vi "SendCmdToSkywire.vi"(6 "wait for response (y)":bool=TRUE, 8 "error in (no error)":errorcluster, 9 "Cmd String":string="AT+CSQ", 10 "Cmd":T1=enum."Send cmd string", 11 "VISA resource name":refnum<visa-resource-name>="COM30") -> (0 "error out":errorcluster, 1 "Response numbers":dbl[](array[numeric])=[5.0, 3.0], 2 "Response string":string="AT+CSQ\r\r\n+CSQ: 5,3\r\n\r\nOK\r\n", 3 "VISA resource name 2":refnum<visa-resource-name>="COM30", 4 "Parsed string response":string, 5 "Parsed string responses":string[](array[string]), 7 "RSSI (dbm)":string="-103")   [LabVIEW 2013]
uses:
  Skywire cmds.ctl
  Test Globals/Global 1.vi
  Main Support/Global 2.vi
panel:
  out "Log resp":string
  out "Msecs to stopped":u32
  out "Msecs to first byte":u32
  out "Bytes at Port":u32=26
  out "timeout":bool
  out "return count":u32=7
  in  "CmdArray":string[](array[string])=["AT+CSQ", "AT+CGMR", "AT+CREG?", "AT+CGREG?", "AT#MEIDESN?", "AT+CGSN", "AT$GPSLOCK?", "In cmd string", "AT", "AT#SIMDET=1", "AT#HDRPS?", "AT+GMM", "AT+KSIMDET=1", "AT#CCID", "AT+CEREG?", "AT+CGMM", "AT+GSN", "AT#SIMDET?"]
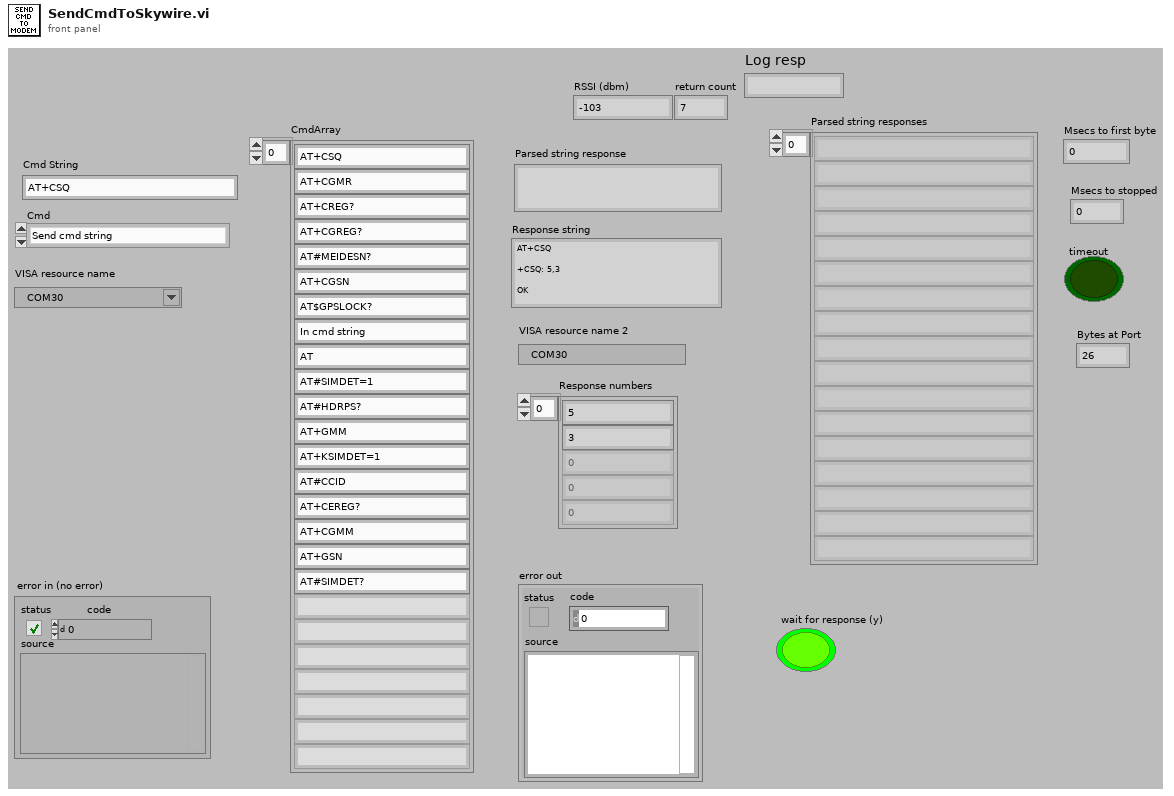
[diagram p1: front panel]
types:
  T1 = typedef "Skywire cmds.ctl" = enum16{"Get primary RSSI", "Get firmware version", "Check 2/3G network reception", "Check LTE network reception", "Get MEID for CDMA", "Get IMEI for 4G/LTE", "Get GPS Coordinates", "Send cmd string", "Check communications", "Enable sim detect", "Check diversity RSSI", "Get make model", "Sierra enable sim det", "get ccid sim id", "Get Gemalto Net Reg", "Get Gemalto model", "Get modem serial number", "Telit sim detect"}
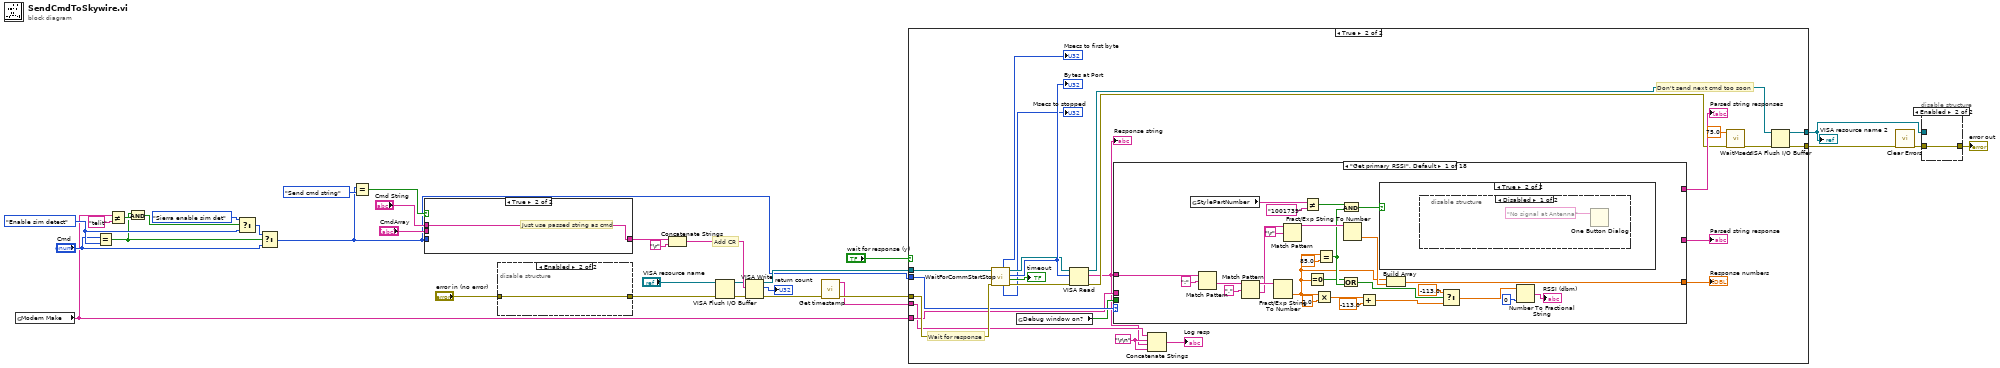
[diagram p0: block diagram]
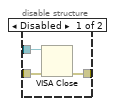
[diagram p2: hidden frame]
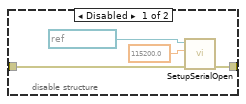
[diagram p3: hidden frame]
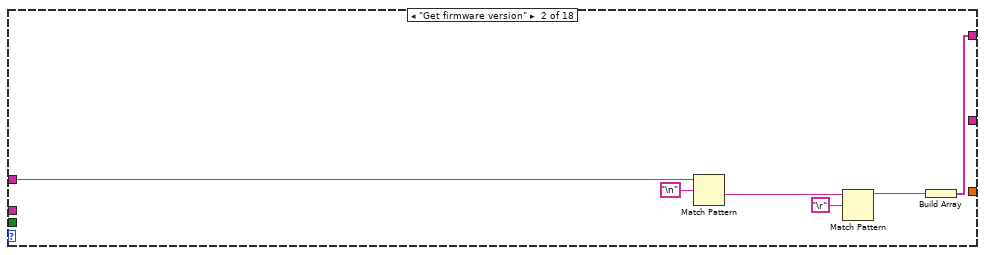
[diagram p7: hidden frame]
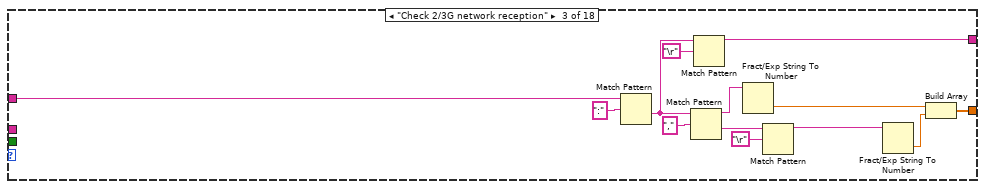
[diagram p8: hidden frame]
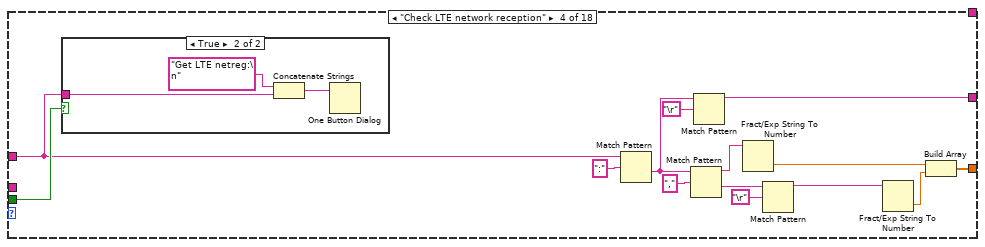
[diagram p9: hidden frame]
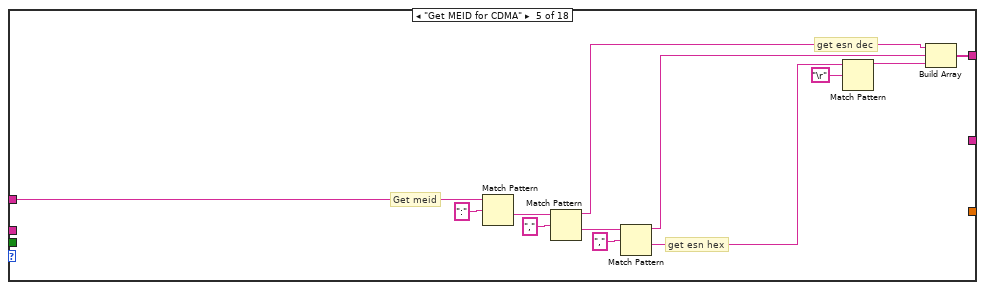
[diagram p11: hidden frame]
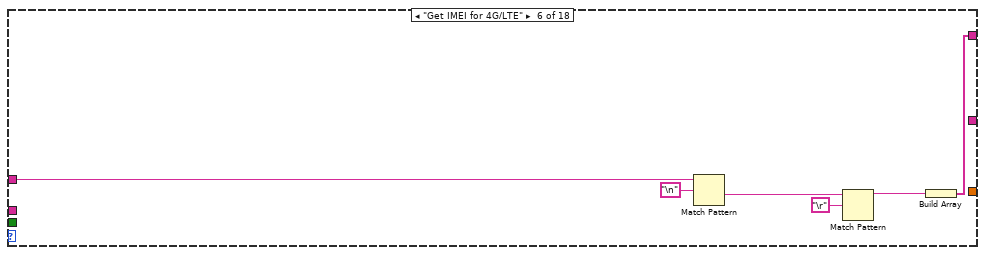
[diagram p12: hidden frame]
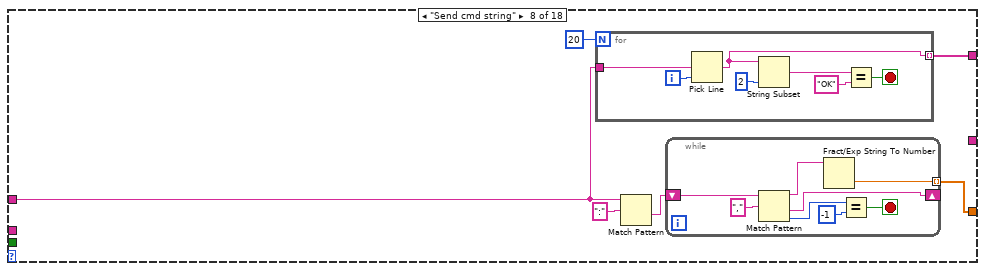
[diagram p14: hidden frame]
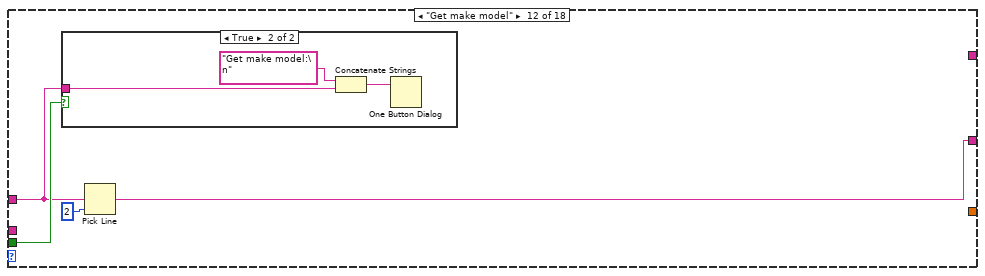
[diagram p18: hidden frame]
diagram:
  w17 = Skywire_cmds."Enable sim detect" ("y")
  # "Add CR"
  n1 = global read "Global 1.vi" "Modem Make"() -> (w4:string)
  n2 = Equal?(x="Cmd", y=w17) -> (x = y?=w15:bool)
  n3 = Not Equal?(x=w4, y="telit") -> (x != y?=w20:bool)
  n4 = And(x=w15, y=w20) -> (x .and. y?=w19:bool)
  n5 = Select(t=Skywire_cmds."Sierra enable sim det" ("y"), s=w19, f=w17) -> (s? t:f=w16:T1)
  n6 = Select(t=w16, s=w15, f="Cmd") -> (s? t:f=w13:T1)
  n7 = Equal?(x=w13, y=Skywire_cmds."Send cmd string") -> (x = y?=w29:bool)
  n8 = case shown="True" w29 {
    tunnel: "CmdArray" -> [w35 _]
    tunnel: [w34 w36] -> w26
    tunnel: "Cmd String" -> [_ w36]
    tunnel: w13 -> [w33 _]
    frame False {
      # "Get cmd string from with cmd as index"
      n9 = Index Array(array=w35, index=w33) -> (element=w34:string)
    }
    frame True {
      # "Just use passed string as cmd"
    }
  }
  n10 = disable-structure shown="Enabled" {
    disable-tunnel: "error in (no error)" -> [w40 w41]
    disable-tunnel: [w39 w41] -> w8
    frame Disabled {
      n11 = call "SetupSerialOpen.vi"("error in (no error)"=w40, "Baud"=115200.0, "VISA Refnum in"=refnum<visa-resource-name> "COM30") -> ("error out"=w39:errorcluster)  [unwired: 7 in, 1 out]
    }
    frame Enabled {
    }
  }
  n12 = Concatenate Strings(w26, "\r") -> (w31:string)
  n13 = VISA Flush I/O Buffer(VISA resource name="VISA resource name", error in (no error)=w8) -> (VISA resource name out=w10:refnum<visa-resource-name>, error out=w12:errorcluster)  [unwired: 1 in]
  n14 = VISA Write(VISA resource name=w10, write buffer=w31, error in (no error)=w12) -> (VISA resource name out=w30:refnum<visa-resource-name>, return count=→"return count":u32, error out=w3:errorcluster)
  n15 = call "Get timestamp.vi"("error in (no error)"=w3) -> ("error out"=w2:errorcluster, "Timestamp"=w1:string)  [unwired: 2 in, 7 out]
  n16 = case shown="True" "wait for response (y)" {
    tunnel: [w43 w54] -> w22
    tunnel: w2 -> [w43 w64]
    tunnel: w30 -> [w42 w63]
    tunnel: w13 -> [_ w60]
    tunnel: [w42 w53] -> w5
    tunnel: w4 -> [_ w48]
    tunnel: w1 -> [_ w47]
    frame False {
    }
    frame True {
      w46 = "\r\n"
      # "Don't send next cmd too soon"
      # "Wait for response"
      n17 = call "WaitForCommStartStop.vi"("error in (no error)"=w64, "VISA Refnum in"=w63) -> ("error out"=w67:errorcluster, "timeout"=→"timeout":bool, "Bytes at Port"=w66:u32, "VISA Refnum out"=w65:refnum<visa-resource-name>, "Msecs to stopped"=→"Msecs to stopped":u32, "Msecs to first byte"=→"Msecs to first byte":u32)  [unwired: 4 in]
      "Bytes at Port" <- w66
      n18 = global read "Global 2.vi" "Debug window on?"() -> (w49:bool)
      n19 = VISA Read(VISA resource name=w65, byte count=w66, error in (no error)=w67) -> (VISA resource name out=w55:refnum<visa-resource-name>, read buffer=w45:string, error out=w56:errorcluster)  [unwired: 1 out]
      "Response string" <- w45
      n20 = case shown="\"Get primary RSSI\", Default" w60 {
        tunnel: w45 -> [w94 w100 w106 w115 w142 w147 _ w151 _ _ _ w171 _ w180 w183 w197 w225 w232]
        tunnel: [w85 _ w105 w120 _ _ _ w153 _ _ _ _ _ _ _ w201 _ _] -> w62
        tunnel: [_ w96 _ _ w132 w144 _ w150 _ _ _ _ _ _ _ _ _ _] -> w61
        tunnel: [_ _ w102 w117 _ _ _ _ _ _ _ w173 _ w178 w187 w194 w227 w233] -> w59
        tunnel: w49 -> [_ _ _ w116 _ _ _ _ _ _ _ w172 _ _ _ _ w226 _]
        tunnel: w48 -> [_ _ _ _ _ _ _ _ _ _ _ _ _ _ _ w200 _ _]
        frame "Get primary RSSI", Default {
          n21 = global read "Global 2.vi" "StylePartNumber"() -> (w77:string)
          n22 = Match Pattern(string=w94, regular expression=":") -> (after substring=w92:string)  [unwired: 1 in, 3 out]
          n23 = Match Pattern(string=w92, regular expression=",") -> (before substring=w90:string, after substring=w89:string)  [unwired: 1 in, 2 out]
          n24 = Fract/Exp String To Number(string=w90) -> (number=w69:dbl)  [unwired: 3 in, 1 out]
          n25 = Match Pattern(string=w89, regular expression="\r") -> (before substring=w87:string)  [unwired: 1 in, 3 out]
          n26 = Not Equal?(x=w77, y="1001739") -> (x != y?=w74:bool)
          n27 = Equal To 0?(x=w69) -> (x = 0?=w71:bool)
          n28 = Multiply(x=w69, y=2.0) -> (x*y=w83:dbl)
          n29 = Equal?(x=w69, y=85.0) -> (x = y?=w72:bool)
          n30 = Or(x=w71, y=w72) -> (x .or. y?=w68:bool)
          n31 = And(x=w74, y=w72) -> (x .and. y?=w73:bool)
          n32 = Fract/Exp String To Number(string=w87) -> (number=w86:dbl)  [unwired: 3 in, 1 out]
          n33 = Add(x=w83, y=-113.0) -> (x+y=w70:dbl)
          n34 = case shown="True" w73 {
            frame False {
            }
            frame True {
              n35 = disable-structure shown="Disabled" {
                frame Disabled {
                  n36 = One Button Dialog(message="No signal at Antenna") -> ()  [unwired: 1 in, 1 out]
                }
                frame Enabled {
                }
              }
            }
          }
          n37 = Build Array(w69, w86) -> (w85:dbl[])
          n38 = Select(t=-113.0, s=w68, f=w70) -> (s? t:f=w78:dbl)
          n39 = Number To Fractional String(number=w78, precision (6)=i16 0) -> (F-format string=→"RSSI (dbm)":string)  [unwired: 2 in]
        }
        frame "Get firmware version" {
          n40 = Match Pattern(string=w100, regular expression="\n") -> (after substring=w101:string)  [unwired: 1 in, 3 out]
          n41 = Match Pattern(string=w101, regular expression="\r") -> (before substring=w97:string)  [unwired: 1 in, 3 out]
          n42 = Build Array(w97) -> (w96:string[])
        }
        frame "Check 2/3G network reception" {
          n43 = Match Pattern(string=w106, regular expression=":") -> (after substring=w103:string)  [unwired: 1 in, 3 out]
          n44 = Match Pattern(string=w103, regular expression=",") -> (before substring=w112:string, after substring=w111:string)  [unwired: 1 in, 2 out]
          n45 = Match Pattern(string=w103, regular expression="\r") -> (before substring=w102:string)  [unwired: 1 in, 3 out]
          n46 = Fract/Exp String To Number(string=w112) -> (number=w108:dbl)  [unwired: 3 in, 1 out]
          n47 = Match Pattern(string=w111, regular expression="\r") -> (before substring=w109:string)  [unwired: 1 in, 3 out]
          n48 = Fract/Exp String To Number(string=w109) -> (number=w107:dbl)  [unwired: 3 in, 1 out]
          n49 = Build Array(w108, w107) -> (w105:dbl[])
        }
        frame "Check LTE network reception" {
          n50 = case shown="True" w116 {
            tunnel: w115 -> [_ w129]
            frame False {
            }
            frame True {
              n51 = Concatenate Strings("Get LTE netreg:\n" ("string"), w129) -> (w130:string)
              n52 = One Button Dialog(message=w130) -> ()  [unwired: 1 in, 1 out]
            }
          }
          n53 = Match Pattern(string=w115, regular expression=":") -> (after substring=w118:string)  [unwired: 1 in, 3 out]
          n54 = Match Pattern(string=w118, regular expression=",") -> (before substring=w126:string, after substring=w125:string)  [unwired: 1 in, 2 out]
          n55 = Match Pattern(string=w118, regular expression="\r") -> (before substring=w117:string)  [unwired: 1 in, 3 out]
          n56 = Fract/Exp String To Number(string=w126) -> (number=w122:dbl)  [unwired: 3 in, 1 out]
          n57 = Match Pattern(string=w125, regular expression="\r") -> (before substring=w123:string)  [unwired: 1 in, 3 out]
          n58 = Fract/Exp String To Number(string=w123) -> (number=w121:dbl)  [unwired: 3 in, 1 out]
          n59 = Build Array(w122, w121) -> (w120:dbl[])
        }
        frame "Get MEID for CDMA" {
          # "get esn hex"
          # "get esn dec"
          # "Get meid"
          n60 = Match Pattern(string=w142, regular expression=":") -> (after substring=w143:string)  [unwired: 1 in, 3 out]
          n61 = Match Pattern(string=w143, regular expression=",") -> (before substring=w137:string, after substring=w138:string)  [unwired: 1 in, 2 out]
          n62 = Match Pattern(string=w138, regular expression=",") -> (before substring=w136:string, after substring=w135:string)  [unwired: 1 in, 2 out]
          n63 = Match Pattern(string=w135, regular expression="\r") -> (before substring=w133:string)  [unwired: 1 in, 3 out]
          n64 = Build Array(w137, w136, w133) -> (w132:string[])
        }
        frame "Get IMEI for 4G/LTE" {
          n65 = Match Pattern(string=w147, regular expression="\n") -> (after substring=w149:string)  [unwired: 1 in, 3 out]
          n66 = Match Pattern(string=w149, regular expression="\r") -> (before substring=w145:string)  [unwired: 1 in, 3 out]
          n67 = Build Array(w145) -> (w144:string[])
        }
        frame "Get GPS Coordinates" {
        }
        frame "Send cmd string" {
          n68 = for {
            N: 20 -> [_]
            tunnel: w151 -> [w162]
            tunnel: [w159] -> w150 mode=indexing
            i -> [w161]
            stop <- w160 stop-if-true
            n69 = Pick Line(multi-line string=w162, line index=w161) -> (output string=w159:string)  [unwired: 1 in]
            n70 = String Subset(string=w159, length (rest)=2 ("length (rest)")) -> (substring=w157:string)  [unwired: 1 in]
            n71 = Equal?(x=w157, y="OK") -> (x = y?=w160:bool)
          }
          n72 = Match Pattern(string=w151, regular expression=":") -> (after substring=w155:string)  [unwired: 1 in, 3 out]
          n73 = while {
            shift-right: [w164] -> _
            shift-left: w155 -> [w168]
            tunnel: [w163] -> w153 mode=indexing
            stop <- w165 stop-if-true
            n74 = Match Pattern(string=w168, regular expression=",") -> (before substring=w170:string, after substring=w164:string, offset past match=w167:i32)  [unwired: 1 in, 1 out]
            n75 = Fract/Exp String To Number(string=w170) -> (number=w163:dbl)  [unwired: 3 in, 1 out]
            n76 = Equal?(x=w167, y=-1) -> (x = y?=w165:bool)
          }
        }
        frame "Check communications" {
        }
        frame "Enable sim detect" {
        }
        frame "Check diversity RSSI" {
        }
        frame "Get make model" {
          n77 = case shown="True" w172 {
            tunnel: w171 -> [_ w175]
            frame False {
            }
            frame True {
              n78 = Concatenate Strings("Get make model:\n" ("string"), w175) -> (w176:string)
              n79 = One Button Dialog(message=w176) -> ()  [unwired: 1 in, 1 out]
            }
          }
          n80 = Pick Line(multi-line string=w171, line index=2) -> (output string=w173:string)  [unwired: 1 in]
        }
        frame "Sierra enable sim det" {
        }
        frame "get ccid sim id" {
          n81 = Match Pattern(string=w180, regular expression="CCID: ") -> (after substring=w179:string)  [unwired: 1 in, 3 out]
          n82 = Match Pattern(string=w179, regular expression="\r") -> (before substring=w178:string)  [unwired: 1 in, 3 out]
        }
        frame "Telit sim detect" {
          n83 = Match Pattern(string=w183, regular expression="SIMDET: ") -> (after substring=w188:string, offset past match=w186:i32)  [unwired: 1 in, 2 out]
          n84 = Equal?(x=w186, y=-1) -> (x = y?=w184:bool)
          n85 = Match Pattern(string=w188, regular expression="\r") -> (before substring=w187:string)  [unwired: 1 in, 3 out]
          n86 = case shown="True" w184 {
            tunnel: w183 -> [_ w191]
            frame False {
            }
            frame True {
              n87 = Concatenate Strings("SIM detect response = " ("string"), w191) -> (w193:string)
              n88 = One Button Dialog(message=w193) -> ()  [unwired: 1 in, 1 out]
            }
          }
        }
        frame "Get Gemalto Net Reg" {
          n89 = Equal?(x=w200, y="wnc") -> (x = y?=w198:bool)
          n90 = case shown="True" w198 {
            tunnel: w197 -> [w206 w219]
            tunnel: [w203 w217] -> w196
            tunnel: [w202 w216] -> w195
            tunnel: [w204 w214] -> w194
            frame False {
              n91 = Match Pattern(string=w206, regular expression=":") -> (after substring=w213:string)  [unwired: 1 in, 3 out]
              n92 = Match Pattern(string=w213, regular expression=",") -> (before substring=w208:string, after substring=w209:string)  [unwired: 1 in, 2 out]
              n93 = Match Pattern(string=w213, regular expression="\r") -> (before substring=w204:string)  [unwired: 1 in, 3 out]
              n94 = Fract/Exp String To Number(string=w208) -> (number=w202:dbl)  [unwired: 3 in, 1 out]
              n95 = Match Pattern(string=w209, regular expression="\r") -> (before substring=w211:string)  [unwired: 1 in, 3 out]
              n96 = Fract/Exp String To Number(string=w211) -> (number=w203:dbl)  [unwired: 3 in, 1 out]
            }
            frame True {
              w218 = "," ("regular expression")
              n97 = Match Pattern(string=w219, regular expression=":") -> (after substring=w224:string)  [unwired: 1 in, 3 out]
              n98 = Match Pattern(string=w224, regular expression=w218) -> (before substring=w220:string, after substring=w221:string)  [unwired: 1 in, 2 out]
              n99 = Match Pattern(string=w224, regular expression="\r") -> (before substring=w214:string)  [unwired: 1 in, 3 out]
              n100 = Fract/Exp String To Number(string=w220) -> (number=w216:dbl)  [unwired: 3 in, 1 out]
              n101 = Match Pattern(string=w221, regular expression=w218) -> (before substring=w222:string)  [unwired: 1 in, 3 out]
              n102 = Fract/Exp String To Number(string=w222) -> (number=w217:dbl)  [unwired: 3 in, 1 out]
            }
          }
          n103 = Build Array(w195, w196) -> (w201:dbl[])
        }
        frame "Get Gemalto model" {
          n104 = case shown="True" w226 {
            tunnel: w225 -> [_ w230]
            frame False {
            }
            frame True {
              n105 = Concatenate Strings("Gemalto model = " ("string"), w230) -> (w229:string)
              n106 = One Button Dialog(message=w229) -> ()  [unwired: 1 in, 1 out]
            }
          }
          n107 = Pick Line(multi-line string=w225, line index=2) -> (output string=w227:string)  [unwired: 1 in]
        }
        frame "Get modem serial number" {
          n108 = Pick Line(multi-line string=w232, line index=2) -> (output string=w233:string)  [unwired: 1 in]
        }
      }
      "Response numbers" <- w62
      "Parsed string response" <- w59
      "Parsed string responses" <- w61
      n109 = Concatenate Strings(w47, w46, w45, w46) -> (→"Log resp":string)
      n110 = call "WaitMsecs.vi"("error in (no error)"=w56, "Wait Msecs"=75.0) -> ("error out"=w58:errorcluster)  [unwired: 9 in]
      n111 = VISA Flush I/O Buffer(VISA resource name=w55, error in (no error)=w58) -> (VISA resource name out=w53:refnum<visa-resource-name>, error out=w54:errorcluster)  [unwired: 1 in]
    }
  }
  "VISA resource name 2" <- w5
  n112 = call <vilib>:"Clear Errors.vi"("error in (no error)"=w22) -> ("error out"=w7:errorcluster)  [unwired: 6 in]
  n113 = disable-structure shown="Enabled" {
    disable-tunnel: w7 -> [w237 w238]
    disable-tunnel: [w236 w238] -> w6
    disable-tunnel: w5 -> [w235 _]
    frame Disabled {
      n114 = VISA Close(VISA resource name=w235, error in (no error)=w237) -> (error out=w236:errorcluster)
    }
    frame Enabled {
    }
  }
  "error out" <- w6
